vi "DebugGlobal.vi"() -> ()   [LabVIEW 2019]
uses:
  <vilib>/vision/Image Controls.llb/IMAQ Image.ctl
panel:
  in  "Spatial Correction Fit Error (camera pixel)":dbl
  in  "Debug Image Update":bool=TRUE
  in  "Mature Tracks Count":i32
  in  "Active Tracks Count":i32
  in  "Completed Tracks #":i32
  in  "Loops Complete":bool
  in  "Draw Stimulus Missed Frames":dbl
  in  "Tracking Missed Frames":dbl
  in  "Camera Missed Frames":dbl
  in  "Camera Buffer Number":u32
  in  "Tracking Rate (Hz)":dbl
  in  "Camera Frame Rate (Hz)":dbl
  in  "Draw Stimulus Frame Rate (Hz)":dbl
  in  "Projector Saving Lag (frames)":i32
  in  "Camera Saving Lag (frames)":i32
  in  "Last Median Filter Updated":string
  in  "Closed Loop Lag (frames)":i32
  in  "median closed loop lag (ms)":dbl
  in  "Stop Reason":string
  in  "Stop Recording":bool
  in  "GUI Refresh Period (ms)":u32=10000
  in  "Debug Track Index":i32
  in  "Debug Image":T1
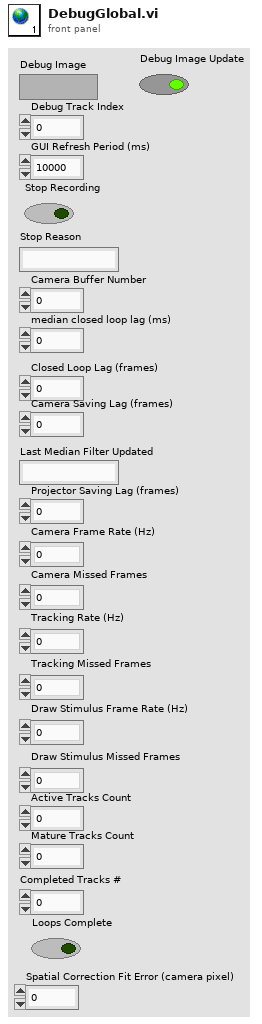
[diagram p1: front panel]
types:
  T1 = typedef "IMAQ Image.ctl" = refnum<image>
diagram:
